vi "Rotation.vi"(1 "Gyro Angle":dbl, 2 "Uncorrected Speed":dbl=-0.0, 3 "Use Correction":bool) -> (0 "Output Speed":dbl=-0.0)   [LabVIEW 2013]
uses:
  Robot Global Data.vi
  <vilib>/addons/control/pid/pid.llb/PID (DBL).vi
  <vilib>/addons/control/pid/NI_PID_pid.lvlib
panel:
  in  "PID gains":T1={"proportional gain (Kc)"=0.015, "integral time (Ti, min)"=0.0, "derivative time (Td, min)"=0.0} {"derivative time (Td, min)" format="%.3f"; "integral time (Ti, min)" format="%.3f"; "proportional gain (Kc)" format="%.3f"}
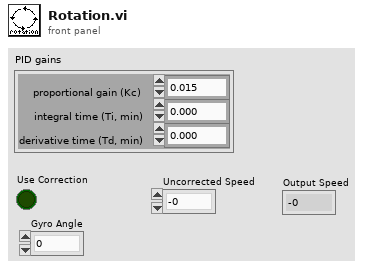
[diagram p1: front panel]
types:
  T1 = cluster{"proportional gain (Kc)":dbl, "integral time (Ti, min)":dbl, "derivative time (Td, min)":dbl}
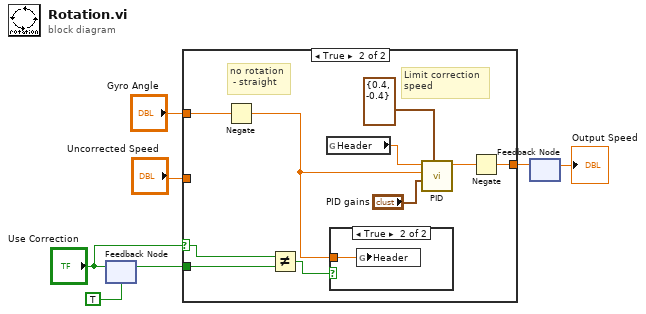
[diagram p0: block diagram]
diagram:
  n1 = feedback #1(TRUE) -> (w7:bool)
  n2 = feedback-in #1("Use Correction") -> ()
  n3 = case shown="True" "Use Correction" {
    selector: "Use Correction" -> [_ w17]
    tunnel: "Uncorrected Speed" -> [w8 _]
    tunnel: [w8 w9] -> w5
    tunnel: w7 -> [_ w18]
    tunnel: "Gyro Angle" -> [_ w11]
    frame False {
    }
    frame True {
      # "Limit correction\nspeed"
      # "no rotation\n - straight"
      n4 = Negate(x=w11) -> (-x=w10:dbl)
      n5 = Not Equal?(x=w17, y=w18) -> (x != y?=w15:bool)
      n6 = global read "Robot Global Data.vi" "Header"() -> (w12:dbl)
      n7 = case shown="True" w15 {
        tunnel: w10 -> [_ w19]
        frame False {
        }
        frame True {
          n8 = global write "Robot Global Data.vi" "Header"(w19) -> ()
        }
      }
      n9 = call-poly <vilib>:"PID.vi"("output range"=cluster{"output high":dbl, "output low":dbl} {"output high"=0.4, "output low"=-0.4}, "PID gains"="PID gains", "process variable"=w10, "setpoint"=w12) -> ("output"=w16:dbl)  [unwired: 2 in, 5 out]
      n10 = Negate(x=w16) -> (-x=w9:dbl)
    }
  }
  n11 = feedback #2() -> (→"Output Speed":dbl)  [unwired: 1 out]
  n12 = feedback-in #2(w5) -> ()
